vi "2Voice.FRAME_RD.vi"(0 "VISA resource name":refnum<visa-resource-name> caption="Serial Port", 1 "baud rate (9600)":u32=9600 caption="波特率(9600)", 2 "timeout(ms)":u32=5000 caption="超时（ms）", 5 "ReadMode":enum16{"0-字符串", "1-字节数组"}(ring), 7 "比较字符串":string, 9 "比较字节数组":u8[](array[numeric]) format="%02x", 11 "error in (no error)":errorcluster caption="错误输入（无错误）", 12 "字节总数":u32) -> (4 "OK?":bool, 8 "读取字符串":string, 10 "读出字节数组":u8[](array[numeric]) format="%02x", 14 "返回数":u32, 15 "error out":errorcluster caption="错误输出")   [LabVIEW 2012, in "Lib_UEL.ATE.lvlib" / "Lib_2Voice.lvlib"]
uses:
  Lib_2Voice.lvlib
  <vilib>/Instr/_visa.llb/VISA Configure Serial Port (Instr).vi
panel:
  # "V001 - Inital Version. ~LI.Guang 2011-05-13"
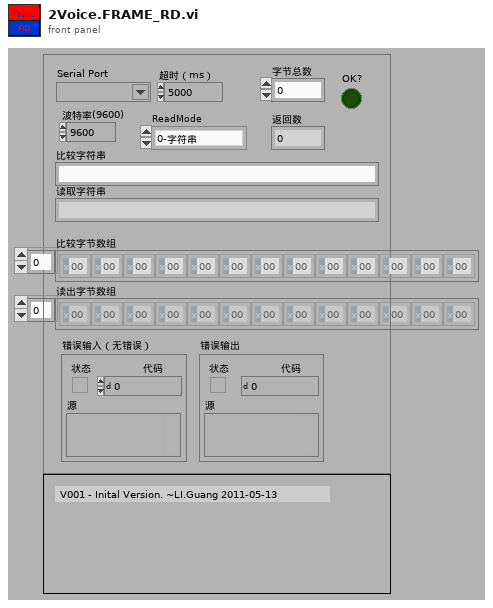
[diagram p1: front panel]
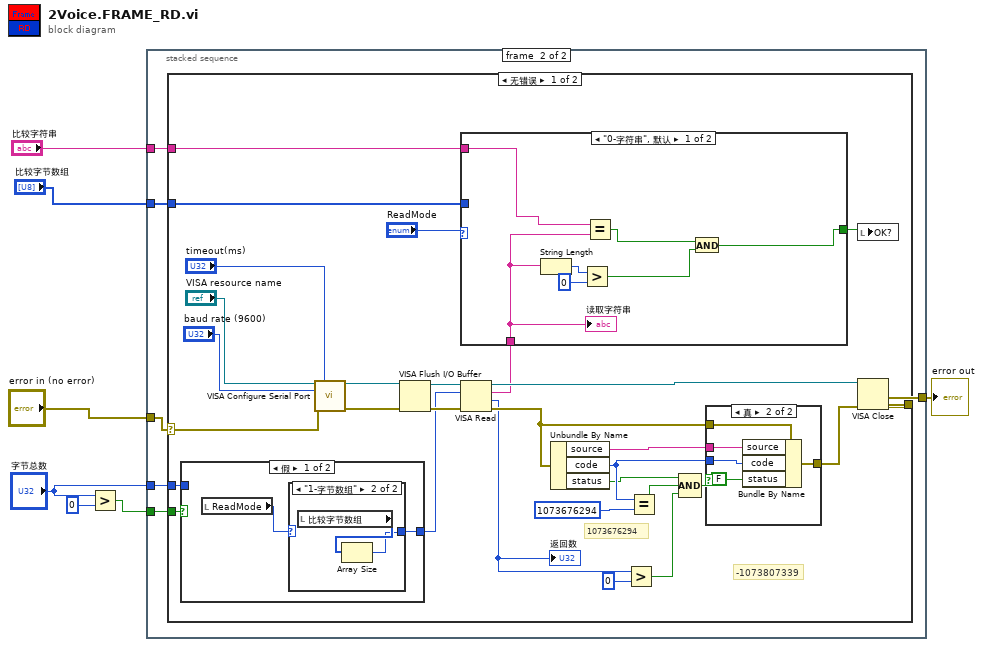
[diagram p0: block diagram]
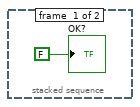
[diagram p2: hidden frame]
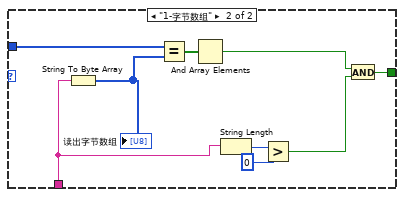
[diagram p3: hidden frame]
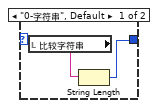
[diagram p4: hidden frame]
diagram:
  n1 = Greater?(x="字节总数", y=u32 0) -> (0:w2:bool)
  n2 = stacked-sequence {
    tunnel: "error in (no error)" -> [_ w14]
    tunnel: [_ w13] -> w6
    tunnel: "比较字节数组" -> [_ w12]
    tunnel: "比较字符串" -> [_ w11]
    tunnel: w2 -> [_ w10]
    tunnel: "字节总数" -> [_ w9]
    frame #0 {
      "OK?" <- FALSE ("OK?")
    }
    frame #1 {
      n3 = case shown="无错误" w14 {
        selector: w14 -> [w40 w73]
        tunnel: [w38 w73] -> w13
        tunnel: w12 -> [w19 _]
        tunnel: w11 -> [w18 _]
        tunnel: w10 -> [w17 _]
        tunnel: w9 -> [w16 _]
        frame No Error {
          # "1073676294"
          # "-1073807339"
          n4 = case shown="假" w17 {
            tunnel: [w60 w66] -> w21
            tunnel: w16 -> [_ w66]
            frame False {
              n5 = local read "ReadMode"() -> (w61:enum16{"0-字符串", "1-字节数组"})
              n6 = case shown="\"1-字节数组\"" w61 {
                tunnel: [w62 w64] -> w60
                frame "0-字符串", Default {
                  n7 = local read "比较字符串"() -> (w63:string)
                  n8 = String Length(string=w63) -> (length=w62:i32)
                }
                frame "1-字节数组" {
                  n9 = local read "比较字节数组"() -> (w65:u8[])
                  n10 = Array Size(array=w65) -> (size(s)=w64:i32)
                }
              }
            }
            frame True {
            }
          }
          n11 = call-poly "VISA Configure Serial Port"("VISA resource name"="VISA resource name", "timeout (10sec)"="timeout(ms)", "baud rate (9600)"="baud rate (9600)", "error in (no error)"=w40) -> ("VISA resource name out"=w37:refnum<visa-resource-name>, "error out"=w36:errorcluster)  [unwired: 10 in]
          n12 = VISA Flush I/O Buffer(VISA resource name=w37, error in (no error)=w36) -> (VISA resource name out=w35:refnum<visa-resource-name>, error out=w34:errorcluster)  [unwired: 1 in]
          n13 = VISA Read(VISA resource name=w35, byte count=w21, error in (no error)=w34) -> (VISA resource name out=w39:refnum<visa-resource-name>, read buffer=w32:string, return count=w24:u32, error out=w31:errorcluster)
          "返回数" <- w24
          n14 = case shown="\"0-字符串\", 默认" "ReadMode" {
            tunnel: w32 -> [w49 w56]
            tunnel: w19 -> [_ w57]
            tunnel: w18 -> [w50 _]
            tunnel: [w44 w51] -> w15
            frame "0-字符串", Default {
              n15 = String Length(string=w49) -> (length=w48:i32)
              n16 = Greater?(x=w48, y=0) -> (0:w45:bool)
              n17 = Equal?(x=w50, y=w49) -> (x = y?=w46:bool)
              n18 = And(x=w46, y=w45) -> (x .and. y?=w44:bool)
              "读取字符串" <- w49
            }
            frame "1-字节数组" {
              n19 = String To Byte Array(string=w56) -> (unsigned byte array=w59:u8[])
              "读出字节数组" <- w59
              n20 = Equal?(x=w57, y=w59) -> (x = y?=w58:bool[])
              n21 = And Array Elements(Boolean array=w58) -> (logical AND=w53:bool)
              n22 = String Length(string=w56) -> (length=w55:i32)
              n23 = Greater?(x=w55, y=0) -> (0:w52:bool)
              n24 = And(x=w53, y=w52) -> (x .and. y?=w51:bool)
            }
          }
          n25 = Unbundle By Name(w31) -> ("source"=w30:string, "code"=w29:i32, "status"=w26:bool)
          n26 = Greater?(x=w24, y=u32 0) -> (0:w22:bool)
          n27 = Equal?(x=w29, y=1073676294) -> (x = y?=w27:bool)
          n28 = Compound Arithmetic op=AND(w26, w27, w22) -> (w25:bool)
          n29 = case shown="真" w25 {
            tunnel: w31 -> [w67 w72]
            tunnel: w30 -> [_ w71]
            tunnel: w29 -> [_ w70]
            tunnel: [w67 w68] -> w28
            frame False {
            }
            frame True {
              n30 = Bundle By Name(cluster=w72, "source"=w71, "code"=w70, "status"=FALSE) -> (w68:errorcluster)
            }
          }
          n31 = local write "OK?"(w15) -> ()
          n32 = VISA Close(VISA resource name=w39, error in (no error)=w28) -> (error out=w38:errorcluster)
        }
        frame Error {
        }
      }
    }
  }
  "error out" <- w6
